vi "ResetAnnotation.vi"(8 "XYG_Up":refnum<vi>, 11 "XYG_Down":refnum<vi>) -> ()   [LabVIEW 2017]
uses:
  <vilib>/Utility/miscctls.llb/LVAnnotationListTypeDef.ctl
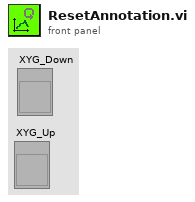
[diagram p1: front panel]
types:
  T1 = typedef "LVAnnotationListTypeDef.ctl" = cluster{"Name":string, "Color":u32, "Style":u8, "Point Style":u8, "Name Visible":bool, "Allow Drag":bool, "Annotation Mode":u32, "Plot":i32, "Index":i32, "Position":cluster{"X":dbl, "Y":dbl}, "X Scale":u32, "Y Scale":u32, "Show Arrow":bool, "Lock Name":bool, "Plot Area":i32, "Label Offset":cluster{"X":dbl, "Y":dbl}}[]
  T2 = cluster{"Annotation List[0]":cluster{"Name":string, "Color":u32, "Style":u8, "Point Style":u8, "Name Visible":bool, "Allow Drag":bool, "Annotation Mode":u32, "Plot":i32, "Index":i32, "Position":cluster{"X":dbl, "Y":dbl}, "X Scale":u32, "Y Scale":u32, "Show Arrow":bool, "Lock Name":bool, "Plot Area":i32, "Label Offset":cluster{"X":dbl, "Y":dbl}}, "Annotation List[1]":cluster{"Name":string, "Color":u32, "Style":u8, "Point Style":u8, "Name Visible":bool, "Allow Drag":bool, "Annotation Mode":u32, "Plot":i32, "Index":i32, "Position":cluster{"X":dbl, "Y":dbl}, "X Scale":u32, "Y Scale":u32, "Show Arrow":bool, "Lock Name":bool, "Plot Area":i32, "Label Offset":cluster{"X":dbl, "Y":dbl}}, "Annotation List[2]":cluster{"Name":string, "Color":u32, "Style":u8, "Point Style":u8, "Name Visible":bool, "Allow Drag":bool, "Annotation Mode":u32, "Plot":i32, "Index":i32, "Position":cluster{"X":dbl, "Y":dbl}, "X Scale":u32, "Y Scale":u32, "Show Arrow":bool, "Lock Name":bool, "Plot Area":i32, "Label Offset":cluster{"X":dbl, "Y":dbl}}, "Annotation List[3]":cluster{"Name":string, "Color":u32, "Style":u8, "Point Style":u8, "Name Visible":bool, "Allow Drag":bool, "Annotation Mode":u32, "Plot":i32, "Index":i32, "Position":cluster{"X":dbl, "Y":dbl}, "X Scale":u32, "Y Scale":u32, "Show Arrow":bool, "Lock Name":bool, "Plot Area":i32, "Label Offset":cluster{"X":dbl, "Y":dbl}}, "Annotation List[4]":cluster{"Name":string, "Color":u32, "Style":u8, "Point Style":u8, "Name Visible":bool, "Allow Drag":bool, "Annotation Mode":u32, "Plot":i32, "Index":i32, "Position":cluster{"X":dbl, "Y":dbl}, "X Scale":u32, "Y Scale":u32, "Show Arrow":bool, "Lock Name":bool, "Plot Area":i32, "Label Offset":cluster{"X":dbl, "Y":dbl}}, "Annotation List[5]":cluster{"Name":string, "Color":u32, "Style":u8, "Point Style":u8, "Name Visible":bool, "Allow Drag":bool, "Annotation Mode":u32, "Plot":i32, "Index":i32, "Position":cluster{"X":dbl, "Y":dbl}, "X Scale":u32, "Y Scale":u32, "Show Arrow":bool, "Lock Name":bool, "Plot Area":i32, "Label Offset":cluster{"X":dbl, "Y":dbl}}, "Annotation List[6]":cluster{"Name":string, "Color":u32, "Style":u8, "Point Style":u8, "Name Visible":bool, "Allow Drag":bool, "Annotation Mode":u32, "Plot":i32, "Index":i32, "Position":cluster{"X":dbl, "Y":dbl}, "X Scale":u32, "Y Scale":u32, "Show Arrow":bool, "Lock Name":bool, "Plot Area":i32, "Label Offset":cluster{"X":dbl, "Y":dbl}}, "Annotation List[7]":cluster{"Name":string, "Color":u32, "Style":u8, "Point Style":u8, "Name Visible":bool, "Allow Drag":bool, "Annotation Mode":u32, "Plot":i32, "Index":i32, "Position":cluster{"X":dbl, "Y":dbl}, "X Scale":u32, "Y Scale":u32, "Show Arrow":bool, "Lock Name":bool, "Plot Area":i32, "Label Offset":cluster{"X":dbl, "Y":dbl}}, "Annotation List[8]":cluster{"Name":string, "Color":u32, "Style":u8, "Point Style":u8, "Name Visible":bool, "Allow Drag":bool, "Annotation Mode":u32, "Plot":i32, "Index":i32, "Position":cluster{"X":dbl, "Y":dbl}, "X Scale":u32, "Y Scale":u32, "Show Arrow":bool, "Lock Name":bool, "Plot Area":i32, "Label Offset":cluster{"X":dbl, "Y":dbl}}}
  T3 = cluster{"Name":string, "Color":u32, "Style":u8, "Point Style":u8, "Name Visible":bool, "Allow Drag":bool, "Annotation Mode":u32, "Plot":i32, "Index":i32, "Position":cluster{"X":dbl, "Y":dbl}, "X Scale":u32, "Y Scale":u32, "Show Arrow":bool, "Lock Name":bool, "Plot Area":i32, "Label Offset":cluster{"X":dbl, "Y":dbl}}[]
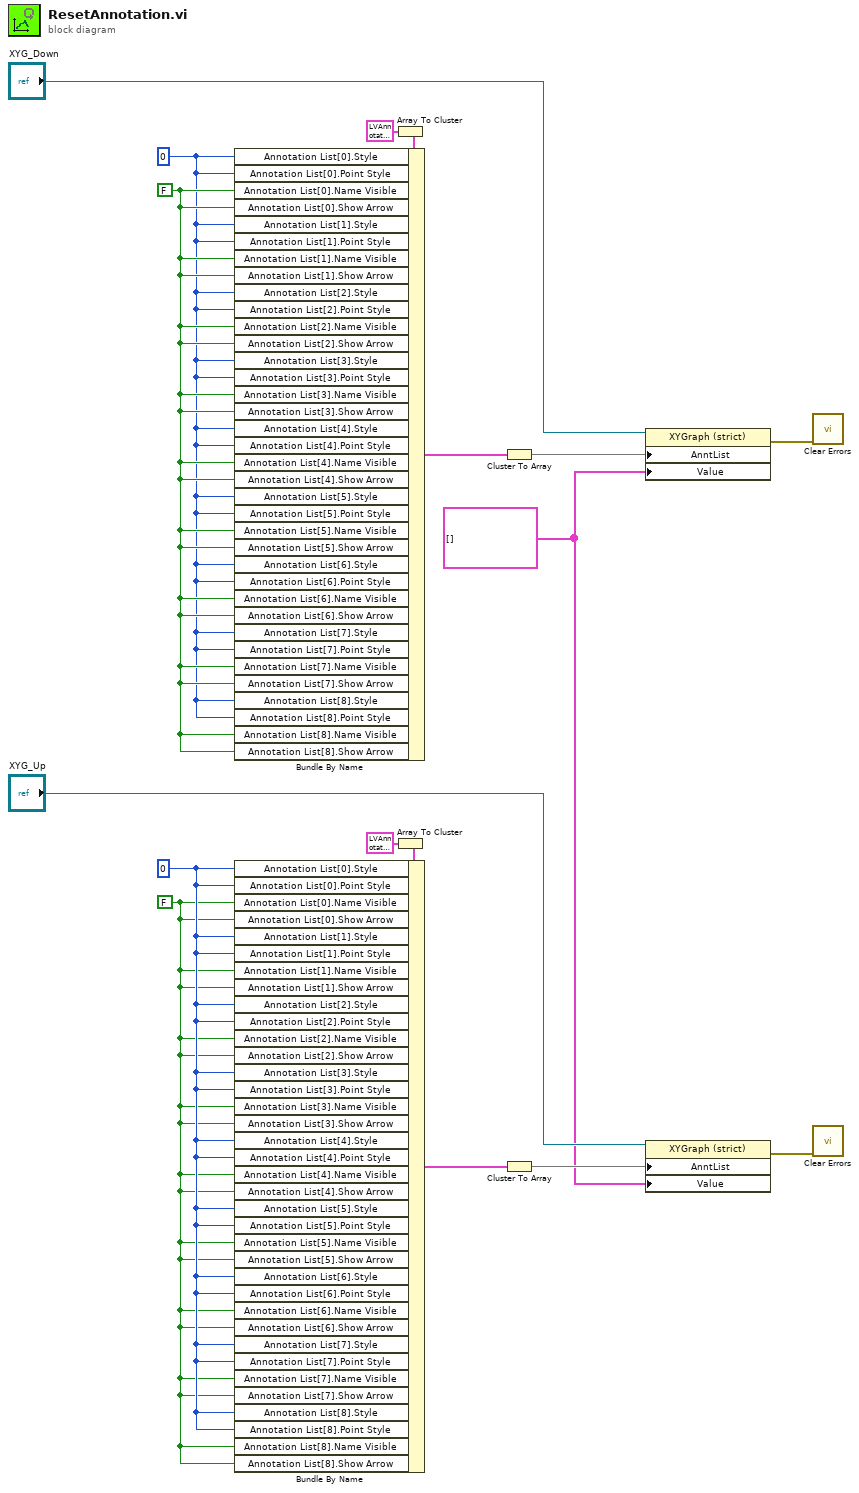
[diagram p0: block diagram]
diagram:
  w2 = FALSE ("Annotation List[0].Name Visible")
  w3 = u8 0 ("Annotation List[0].Style")
  w1 = cluster{"Y":dbl[], "Y":dbl[]}[] [] ("Value")
  w17 = FALSE ("Annotation List[0].Name Visible")
  w16 = u8 0 ("Annotation List[0].Style")
  n1 = Array To Cluster(array=T1 [{"Name"="", "Color"=0, "Style"=0, "Point Style"=0, "Name Visible"=FALSE, "Allow Drag"=FALSE, "Annotation Mode"=0, "Plot"=0, "Index"=0, "Position"={"X"=0.0, "Y"=0.0}, "X Scale"=0, "Y Scale"=0, "Show Arrow"=FALSE, "Lock Name"=FALSE, "Plot Area"=0, "Label Offset"={"X"=0.0, "Y"=0.0}}] ("Annotation List")) -> (cluster=w11:T2)
  n2 = Bundle By Name(cluster=w11, "Annotation List[0].Style"=w16, "Annotation List[0].Point Style"=w16, "Annotation List[0].Name Visible"=w17, "Annotation List[0].Show Arrow"=w17, "Annotation List[1].Style"=w16, "Annotation List[1].Point Style"=w16, "Annotation List[1].Name Visible"=w17, "Annotation List[1].Show Arrow"=w17, "Annotation List[2].Style"=w16, "Annotation List[2].Point Style"=w16, "Annotation List[2].Name Visible"=w17, "Annotation List[2].Show Arrow"=w17, "Annotation List[3].Style"=w16, "Annotation List[3].Point Style"=w16, "Annotation List[3].Name Visible"=w17, "Annotation List[3].Show Arrow"=w17, "Annotation List[4].Style"=w16, "Annotation List[4].Point Style"=w16, "Annotation List[4].Name Visible"=w17, "Annotation List[4].Show Arrow"=w17, "Annotation List[5].Style"=w16, "Annotation List[5].Point Style"=w16, "Annotation List[5].Name Visible"=w17, "Annotation List[5].Show Arrow"=w17, "Annotation List[6].Style"=w16, "Annotation List[6].Point Style"=w16, "Annotation List[6].Name Visible"=w17, "Annotation List[6].Show Arrow"=w17, "Annotation List[7].Style"=w16, "Annotation List[7].Point Style"=w16, "Annotation List[7].Name Visible"=w17, "Annotation List[7].Show Arrow"=w17, "Annotation List[8].Style"=w16, "Annotation List[8].Point Style"=w16, "Annotation List[8].Name Visible"=w17, "Annotation List[8].Show Arrow"=w17) -> (w12:T2)
  n3 = Array To Cluster(array=T1 [{"Name"="", "Color"=0, "Style"=0, "Point Style"=0, "Name Visible"=FALSE, "Allow Drag"=FALSE, "Annotation Mode"=0, "Plot"=0, "Index"=0, "Position"={"X"=0.0, "Y"=0.0}, "X Scale"=0, "Y Scale"=0, "Show Arrow"=FALSE, "Lock Name"=FALSE, "Plot Area"=0, "Label Offset"={"X"=0.0, "Y"=0.0}}] ("Annotation List")) -> (cluster=w8:T2)
  n4 = Bundle By Name(cluster=w8, "Annotation List[0].Style"=w3, "Annotation List[0].Point Style"=w3, "Annotation List[0].Name Visible"=w2, "Annotation List[0].Show Arrow"=w2, "Annotation List[1].Style"=w3, "Annotation List[1].Point Style"=w3, "Annotation List[1].Name Visible"=w2, "Annotation List[1].Show Arrow"=w2, "Annotation List[2].Style"=w3, "Annotation List[2].Point Style"=w3, "Annotation List[2].Name Visible"=w2, "Annotation List[2].Show Arrow"=w2, "Annotation List[3].Style"=w3, "Annotation List[3].Point Style"=w3, "Annotation List[3].Name Visible"=w2, "Annotation List[3].Show Arrow"=w2, "Annotation List[4].Style"=w3, "Annotation List[4].Point Style"=w3, "Annotation List[4].Name Visible"=w2, "Annotation List[4].Show Arrow"=w2, "Annotation List[5].Style"=w3, "Annotation List[5].Point Style"=w3, "Annotation List[5].Name Visible"=w2, "Annotation List[5].Show Arrow"=w2, "Annotation List[6].Style"=w3, "Annotation List[6].Point Style"=w3, "Annotation List[6].Name Visible"=w2, "Annotation List[6].Show Arrow"=w2, "Annotation List[7].Style"=w3, "Annotation List[7].Point Style"=w3, "Annotation List[7].Name Visible"=w2, "Annotation List[7].Show Arrow"=w2, "Annotation List[8].Style"=w3, "Annotation List[8].Point Style"=w3, "Annotation List[8].Name Visible"=w2, "Annotation List[8].Show Arrow"=w2) -> (w7:T2)
  n5 = Cluster To Array(cluster=w12) -> (array=w13:T3)
  n6 = Cluster To Array(cluster=w7) -> (array=w6:T3)
  n7 = property class="XYGraph (strict)"(reference="XYG_Down", "AnntList"=w13, "Value"=w1) -> (error out=w15:errorcluster)  [unwired: 1 in, 1 out]
  n8 = property class="XYGraph (strict)"(reference="XYG_Up", "AnntList"=w6, "Value"=w1) -> (error out=w4:errorcluster)  [unwired: 1 in, 1 out]
  n9 = call <vilib>:"Clear Errors.vi"("error in (no error)"=w15) -> ()  [unwired: 5 in, 2 out]
  n10 = call <vilib>:"Clear Errors.vi"("error in (no error)"=w4) -> ()  [unwired: 5 in, 2 out]
